vi "Charge Test Bench.vi"() -> ()   [LabVIEW 2014]
uses:
  Controls/Current Limit Output.ctl
  Controls/Gen Data.ctl
  Controls/StringSelector.ctl
  Controls/ES System Data.ctl
  Controls/FPGA Data.ctl
panel:
  out "String 2":string
  in  "Gen East Faults (30075-30099)":i16[](array[numeric])
  in  "Gen West Faults (30060-30074)":i16[](array[numeric])
  out "String":string
  out "Frequency Setpoint":sgl
  out "Current Setpoint":dbl
  out "Exit Charge Mode":bool
  out "PV Control":bool
  out "Error Out":errorcluster
  in  "Error In":errorcluster
  in  "FPGA Data":T1 {"SSG Active Current" format="%2.1f"; "PV Reactive Power (L1)" format="%2.1f"; "PV Reactive Power (L2)" format="%2.1f"; "PV Total Reactive Power" format="%2.1f"; "Gen Reactive Power (L1)" format="%2.1f"; "Gen Reactive Power (L2)" format="%2.1f"; "Gen Total Reactive Power" format="%2.1f"; "SSG Reactive Power (L1)" format="%2.1f"; "SSG Reactive Power (L2)" format="%2.1f"; "SSG Total Reactive Power" format="%2.1f"; "PV Total Current" format="%2.1f"; "PV Total Voltage" format="%2.1f"; "PV Active Power (L1)" format="%2.1f"; "PV Active Power (L2)" format="%2.1f"; "PV App Power (L1)" format="%2.1f"; "PV App Power (L2)" format="%2.1f"; "PV Total Active Power" format="%2.1f"; "PV Total App Power" format="%2.1f"; "PV Arms (L1)" format="%2.1f"; "PV Arms (L2)" format="%2.1f"; "PV Vrms (L1)" format="%2.1f"; "PV Vrms (L2)" format="%2.1f"; "Gen Total Current" format="%2.1f"; "SSG Total Current" format="%2.1f"; "Gen Total Voltage" format="%2.1f"; "SSG Total Voltage" format="%2.1f"; "Gen Active Power (L1)" format="%2.1f"; "Gen Active Power (L2)" format="%2.1f"; "SSG Active Power (L1)" format="%2.1f"; "SSG Active Power (L2)" format="%2.1f"; "Gen App Power (L1)" format="%2.1f"; "Gen App Power (L2)" format="%2.1f"; "SSG App Power (L1)" format="%2.1f"; "SSG App Power (L2)" format="%2.1f"; "Gen Total Active Power" format="%2.1f"; "Gen Total App Power" format="%2.1f"; "Gen Arms (L1)" format="%2.1f"; "Gen Arms (L2)" format="%2.1f"; "Gen Vrms (L1)" format="%2.1f"; "Gen Vrms (L2)" format="%2.1f"; "SSG Total Active Power" format="%2.1f"; "SSG Total App Power" format="%2.1f"; "SSG Arms (L1)" format="%2.1f"; "SSG Arms (L2)" format="%2.1f"; "SSG Vrms (L1)" format="%2.1f"; "SSG Vrms (L2)" format="%2.1f"}
  in  "ES System Data":T2={"Voltage"=0.0, "Current"=0.0, "SOC Avg"=0.0, "Faults"=0, "Alarms"=0, "# Strings"=0, "Max Temp"=0, "Min Temp"=0, "Max Cell Voltage"=0.0, "Min Cell Voltage"=0.0, "Energy Capacity"=0.0, "Energy Remaining"=0.0, "SOC Min"=0.0, "SOC Max"=0.0, "ES Fault"=FALSE, "String Select"=enum."3 Strings", "ES Com Fault"=FALSE, "SOH Avg"=0.0}
  in  "Gen Data":T4 {"Alarms" format="%04x"}
  in  "Current Limit Output":T5
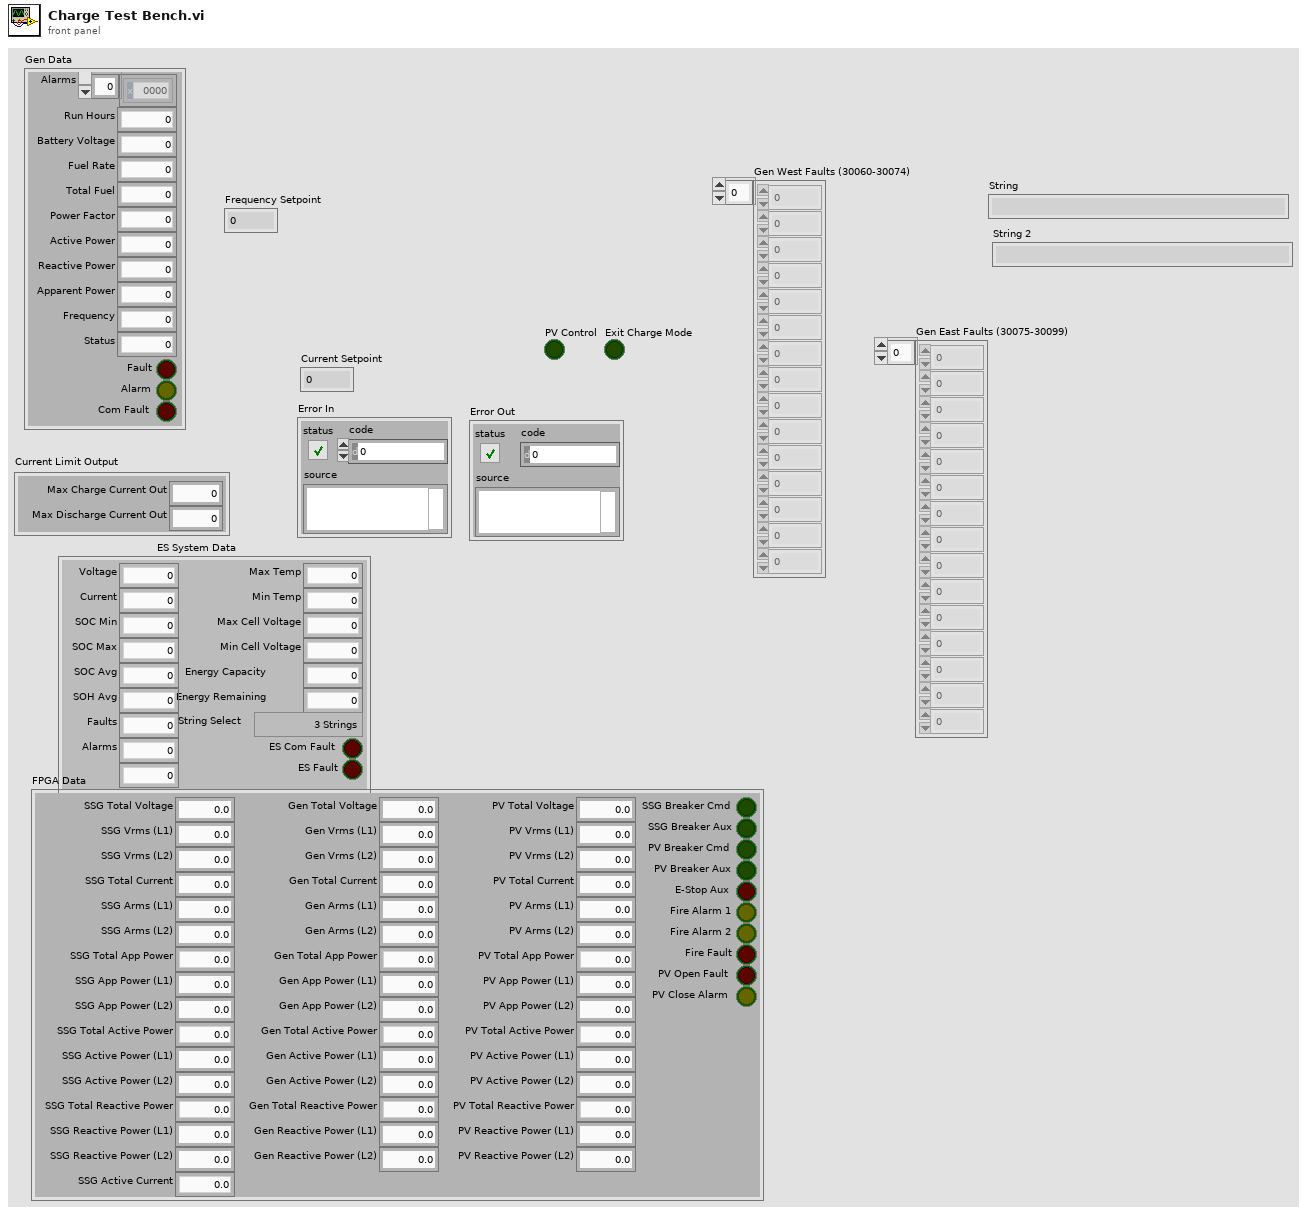
[diagram p1: front panel]
types:
  T1 = typedef "FPGA Data.ctl" = cluster{"Gen Total Voltage":dbl, "Gen Vrms (L1)":dbl, "Gen Vrms (L2)":dbl, "Gen Total Current":dbl, "Gen Arms (L1)":dbl, "Gen Arms (L2)":dbl, "Gen Total App Power":dbl, "Gen App Power (L1)":dbl, "Gen App Power (L2)":dbl, "Gen Total Active Power":dbl, "Gen Active Power (L1)":dbl, "Gen Active Power (L2)":dbl, "Gen Total Reactive Power":dbl, "Gen Reactive Power (L1)":dbl, "Gen Reactive Power (L2)":dbl, "SSG Total Voltage":dbl, "SSG Vrms (L1)":dbl, "SSG Vrms (L2)":dbl, "SSG Total Current":dbl, "SSG Arms (L1)":dbl, "SSG Arms (L2)":dbl, "SSG Total App Power":dbl, "SSG App Power (L1)":dbl, "SSG App Power (L2)":dbl, "SSG Total Active Power":dbl, "SSG Active Power (L1)":dbl, "SSG Active Power (L2)":dbl, "SSG Total Reactive Power":dbl, "SSG Reactive Power (L1)":dbl, "SSG Reactive Power (L2)":dbl, "PV Total Voltage":dbl, "PV Vrms (L1)":dbl, "PV Vrms (L2)":dbl, "PV Total Current":dbl, "PV Arms (L1)":dbl, "PV Arms (L2)":dbl, "PV Total App Power":dbl, "PV App Power (L1)":dbl, "PV App Power (L2)":dbl, "PV Total Active Power":dbl, "PV Active Power (L1)":dbl, "PV Active Power (L2)":dbl, "PV Total Reactive Power":dbl, "PV Reactive Power (L1)":dbl, "PV Reactive Power (L2)":dbl, "SSG Breaker Cmd":bool, "SSG Breaker Aux":bool, "PV Breaker Cmd":bool, "PV Breaker Aux":bool, "E-Stop Aux":bool, "Fire Alarm 1":bool, "Fire Alarm 2":bool, "Fire Fault":bool, "PV Open Fault":bool, "PV Close Alarm":bool, "SSG Active Current":dbl}
  T2 = typedef "ES System Data.ctl" = cluster{"Voltage":sgl, "Current":sgl, "SOC Avg":sgl, "Faults":u16, "Alarms":u16, "# Strings":u16, "Max Temp":i16, "Min Temp":i16, "Max Cell Voltage":sgl, "Min Cell Voltage":sgl, "Energy Capacity":sgl, "Energy Remaining":sgl, "SOC Min":sgl, "SOC Max":sgl, "ES Fault":bool, "String Select":T3, "ES Com Fault":bool, "SOH Avg":sgl}
  T3 = typedef "StringSelector.ctl" = enum16{"1 String (1)", "1 String (2)", "1 String (3)", "2 Strings (1 2)", "2 Strings (2 3)", "2 Strings (1 3)", "3 Strings"}
  T4 = typedef "Gen Data.ctl" = cluster{"Alarms":i16[], "Run Hours":dbl, "Battery Voltage":dbl, "Fuel Rate":dbl, "Total Fuel":dbl, "Power Factor":dbl, "Active Power":dbl, "Reactive Power":dbl, "Apparent Power":dbl, "Frequency":dbl, "Status":u16, "Fault":bool, "Alarm":bool, "Com Fault":bool}
  T5 = typedef "Current Limit Output.ctl" = cluster{"Max Charge Current Out":dbl, "Max Discharge Current Out":dbl}
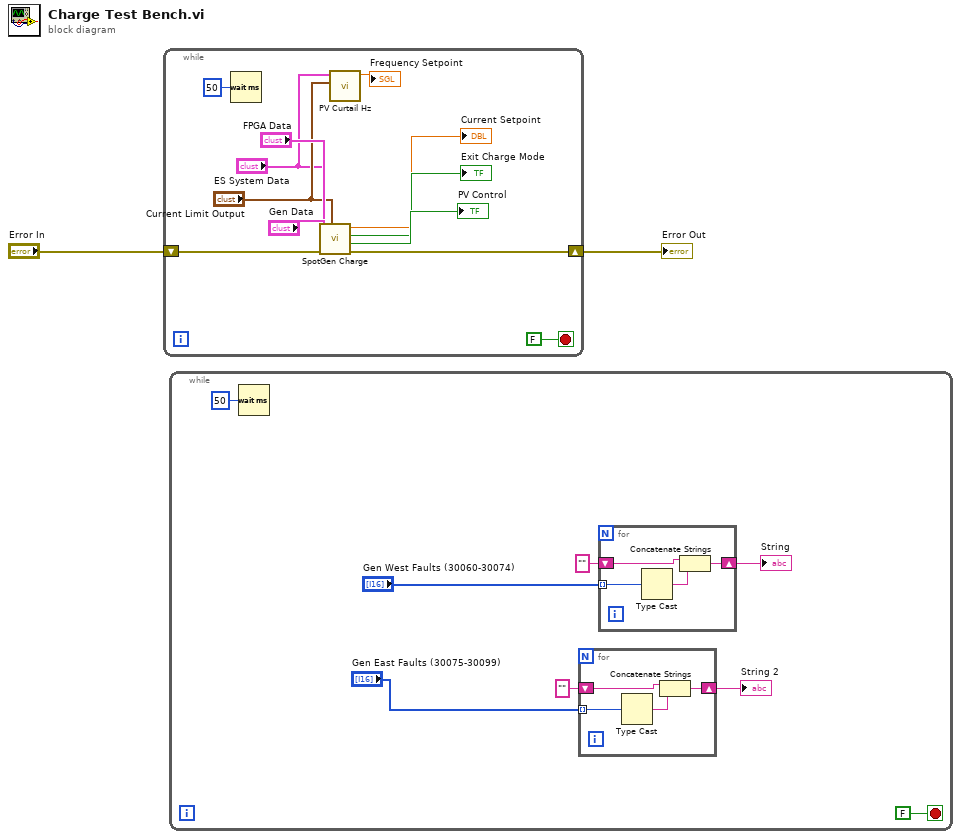
[diagram p0: block diagram]
diagram:
  n1 = while {
    shift-right: [w12] -> w1
    shift-left: "Error In" -> [w13]
    stop <- FALSE stop-if-true
    n2 = Wait (ms)(milliseconds to wait=u32 50) -> ()  [unwired: 1 out]
    n3 = call "SpotGen Charge.vi"("Init"="Current Limit Output", "Error In"=w13, "FPGA Data"="FPGA Data", "ES System Data"="ES System Data", 11:"Gen Data") -> ("Error Out"=w12:errorcluster, "PV Control"=→"PV Control":bool, "Exit Charge Mode"=→"Exit Charge Mode":bool, "Current Setpoint"=→"Current Setpoint":dbl)  [unwired: 3 in]
    n4 = call "PV Curtail Hz.vi"("Current Limit Output"="Current Limit Output", "FPGA Data"="ES System Data") -> ("Frequency Setpoint"=→"Frequency Setpoint":sgl)  [unwired: 8 in, 1 out]
  }
  "Error Out" <- w1
  n5 = while {
    stop <- FALSE stop-if-true
    n6 = Wait (ms)(milliseconds to wait=u32 50) -> ()  [unwired: 1 out]
    n7 = for {
      tunnel: "Gen East Faults (30075-30099)" -> [w26] mode=indexing
      shift-right: [w25] -> w17
      shift-left: "" -> [w23]
      n8 = Type Cast(x=w26) -> (*(type *) &x=w24:string)  [unwired: 1 in]
      n9 = Concatenate Strings(w23, w24) -> (w25:string)
    }
    "String 2" <- w17
    n10 = for {
      tunnel: "Gen West Faults (30060-30074)" -> [w30] mode=indexing
      shift-right: [w29] -> w22
      shift-left: "" -> [w27]
      n11 = Type Cast(x=w30) -> (*(type *) &x=w28:string)  [unwired: 1 in]
      n12 = Concatenate Strings(w27, w28) -> (w29:string)
    }
    "String" <- w22
  }
